vi "Properties to Property Info_2.vi"(6 "Class":string, 7 "Action":T1, 8 "Error In":errorcluster, 11 "All Properties for Refnum Terminal":T3(array[cluster])) -> (0 "Error Out":errorcluster, 2 "Properties for Tree Out":T2(array[cluster]), 3 "Property Info Array":T4(array[cluster]))   [LabVIEW 2023]
doc: "Take properties as returned by LabVIEW property node, and compile property info from property description file.\n\nThis version works for dialogs where you want to show the properties currently displayed in a node.e"
uses:
  controls/action enum.ctl
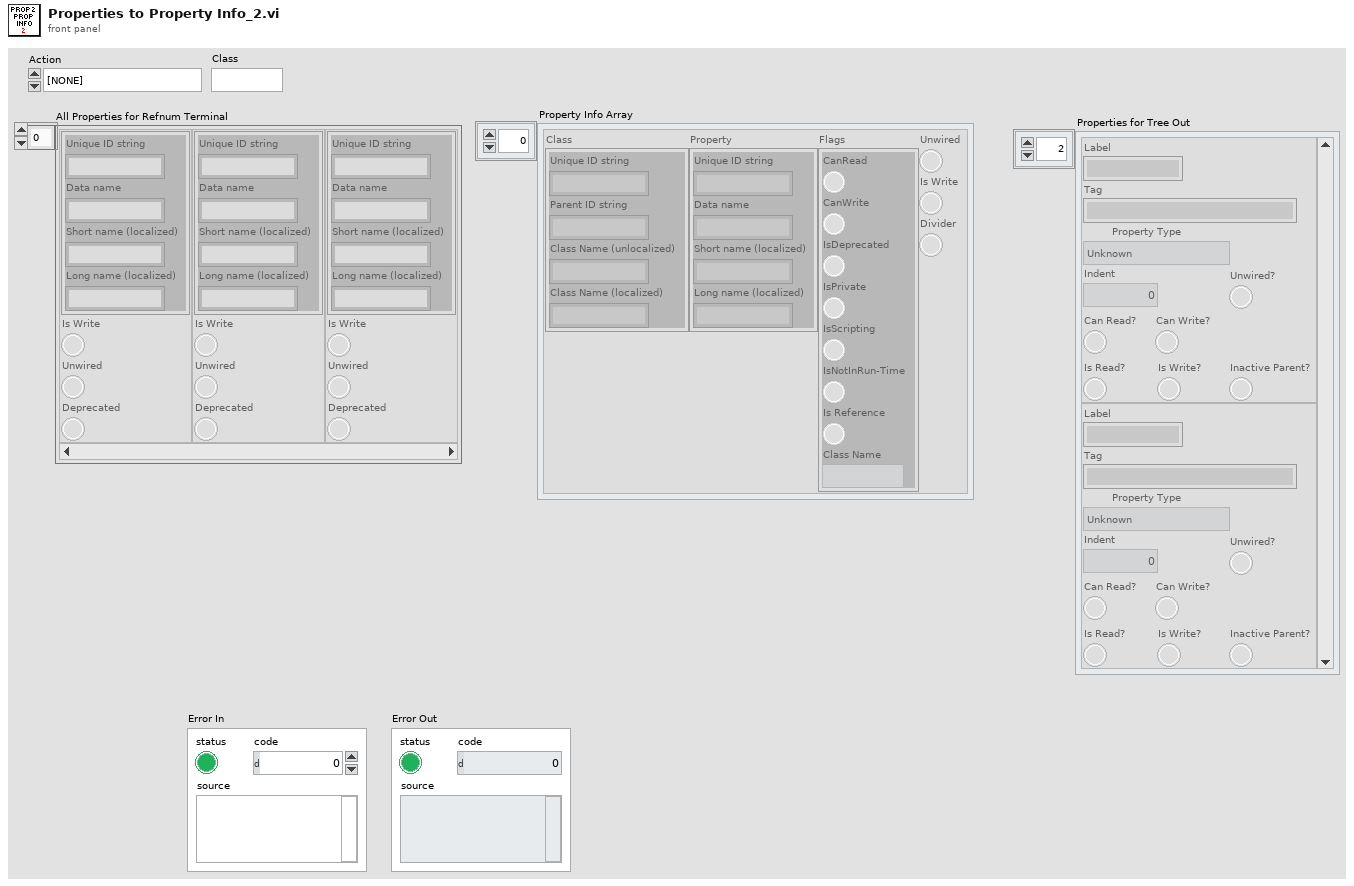
[diagram p1: front panel]
types:
  T1 = typedef "action enum.ctl" = enum16{"[NONE]", "Wire Bundle", "Wire Unbundle", "Terminal Unbundle", "Terminal Bundle", "Bundler Move Up", "Bundler Move Down", "Bundler Insert", "Bundler Remove", "Bundler Remove Unwired", "Bundler Rearrange", "In Place Insert", "In Place Remove", "In Place Remove Unwired", "In Place Rearrange", "Wire Properties", "Wire Method", "Terminal Properties", "Terminal Method", "Property Move Up", "Property Move Down", "Properties Insert", "Properties Remove", "Properties Remove Unwired", "Properties Rearrange", "Method Change", "Class for Constant", "Class For Control", "Class For Node", "Class Name to Clipboard"}
  T2 = cluster{"Label":string, "Tag":string, "Property Type":enum16{"Unknown", "Base", "Scripting", "Private", "Deprecated", "None", "Divider"}, "Indent":u16, "Can Read?":bool, "Can Write?":bool, "Is Read?":bool, "Is Write?":bool, "Inactive Parent?":bool, "Unwired?":bool}[]
  T3 = cluster{"Property/Method Info":cluster{"Unique ID string":string, "Data name":string, "Short name (localized)":string, "Long name (localized)":string}, "Is Write":bool, "Unwired":bool, "Deprecated":bool}[]
  T4 = cluster{"Class":cluster{"Unique ID string":string, "Parent ID string":string, "Class Name (unlocalized)":string, "Class Name (localized)":string}, "Property":cluster{"Unique ID string":string, "Data name":string, "Short name (localized)":string, "Long name (localized)":string}, "Flags":cluster{"CanRead":bool, "CanWrite":bool, "IsDeprecated":bool, "IsPrivate":bool, "IsScripting":bool, "IsNotInRun-Time":bool, "Is Reference":bool, "Class Name":string}, "Divider":bool, "Is Write":bool, "Unwired":bool}[]
  T5 = cluster{"Undotted Property":string, "Bare Property":string, "Is dotted?":bool, "Dot depth":i32, "Indent":i32, "Property Hierarchy":string[], "Parents":string[]}
  T6 = cluster{"Unique ID string":string, "Data name":string, "Short name (localized)":string, "Long name (localized)":string}
  T7 = cluster{"Class":cluster{"Unique ID string":string, "Parent ID string":string, "Class Name (unlocalized)":string, "Class Name (localized)":string}, "Property":cluster{"Unique ID string":string, "Data name":string, "Short name (localized)":string, "Long name (localized)":string}, "Flags":cluster{"CanRead":bool, "CanWrite":bool, "IsDeprecated":bool, "IsPrivate":bool, "IsScripting":bool, "IsNotInRun-Time":bool, "Is Reference":bool, "Class Name":string}, "Divider":bool, "Is Write":bool, "Unwired":bool}
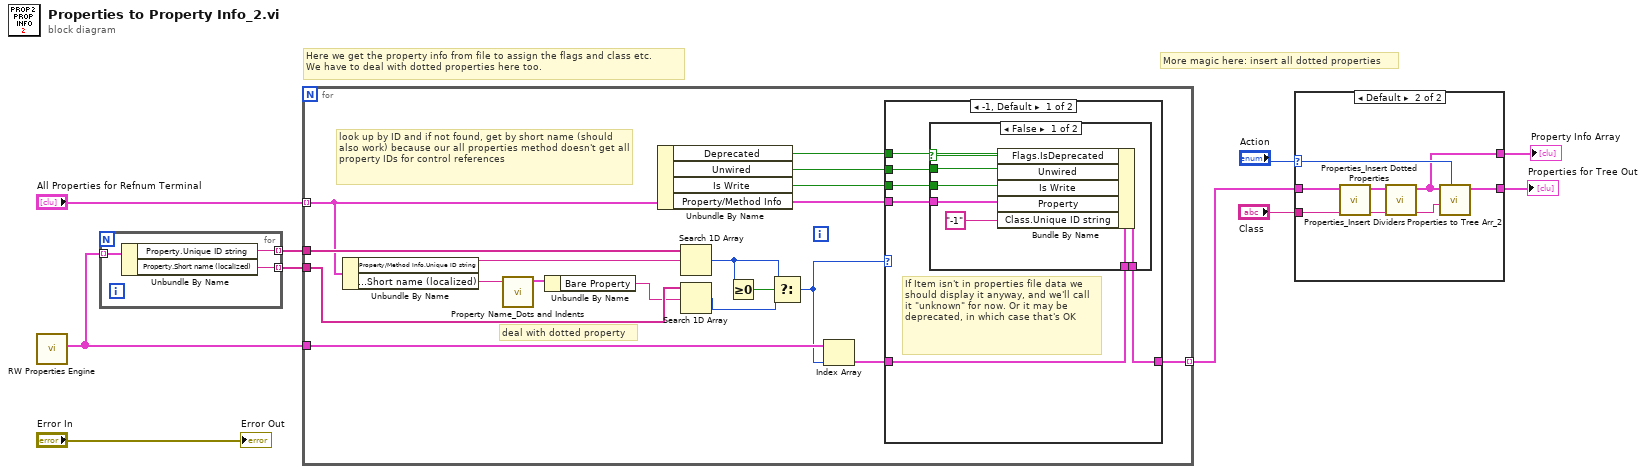
[diagram p0: block diagram]
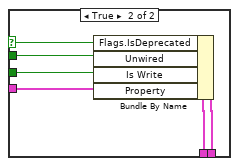
[diagram p2: hidden frame]
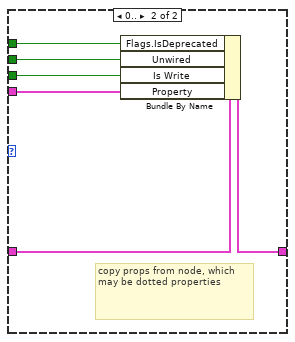
[diagram p3: hidden frame]
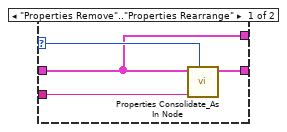
[diagram p4: hidden frame]
diagram:
  # "More magic here: insert all dotted properties"
  # "Here we get the property info from file to assign the flags and class etc. \nWe have to deal with dotted properties here too."
  n1 = call "RW Properties Engine.vi"() -> ("Properties Out"=w10:T4)  [unwired: 7 in, 4 out]
  n2 = for {
    tunnel: w10 -> [w13] mode=indexing
    tunnel: [w12] -> w8 mode=indexing
    tunnel: [w11] -> w7 mode=indexing
    n3 = Unbundle By Name(w13) -> ("Property.Unique ID string"=w12:string, "Property.Short name (localized)"=w11:string)
  }
  n4 = for {
    tunnel: w8 -> [w31]
    tunnel: "All Properties for Refnum Terminal" -> [w14] mode=indexing
    tunnel: w10 -> [w29]
    tunnel: [w27] -> w2 mode=indexing
    tunnel: w7 -> [w26]
    # "deal with dotted property"
    # "look up by ID and if not found, get by short name (should also work) because our all properties method doesn't get all property IDs for control references"
    n5 = Unbundle By Name(w14) -> ("Property/Method Info.Unique ID string"=w30:string, "Property/Method Info.Short name (localized)"=w21:string)
    n6 = call "Property Name_Dots and Indents.vi"("Property"=w21) -> ("Cluster"=w20:T5)  [unwired: 10 in]
    n7 = Unbundle By Name(w20) -> ("Bare Property"=w19:string)
    n8 = Unbundle By Name(w14) -> ("Deprecated"=w15:bool, "Unwired"=w17:bool, "Is Write"=w16:bool, "Property/Method Info"=w18:T6)
    n9 = Search 1D Array(1D array=w31, element=w30) -> (index of element=w23:i32)  [unwired: 1 in]
    n10 = Search 1D Array(1D array=w26, element=w19) -> (index of element=w24:i32)  [unwired: 1 in]
    n11 = Greater Or Equal To 0?(x=w23) -> (x >= 0?=w25:bool)
    n12 = Select(t=w23, s=w25, f=w24) -> (s? t:f=w22:i32)
    n13 = Index Array(array=w29, index=w22) -> (element=w28:T7)
    n14 = case shown="-1, Default" w22 {
      tunnel: [w37 w56] -> w27
      tunnel: w28 -> [w34 w55]
      tunnel: w18 -> [w33 w54]
      tunnel: w17 -> [w36 w53]
      tunnel: w16 -> [w35 w52]
      tunnel: w15 -> [w32 w51]
      frame -1, Default {
        # "If Item isn't in properties file data we should display it anyway, and we'll call it \"unknown\" for now. Or it may be deprecated, in which case that's OK"
        n15 = case shown="False" w32 {
          selector: w32 -> [w38 w45]
          tunnel: [w44 w50] -> w37
          tunnel: w36 -> [w43 w49]
          tunnel: w35 -> [w42 w48]
          tunnel: w34 -> [w41 w47]
          tunnel: w33 -> [w40 w46]
          frame False {
            n16 = Bundle By Name(cluster=w41, "Flags.IsDeprecated"=w38, "Unwired"=w43, "Is Write"=w42, "Property"=w40, "Class.Unique ID string"="-1" ("Class Info.Unique ID string")) -> (w44:T7)
          }
          frame True {
            n17 = Bundle By Name(cluster=w47, "Flags.IsDeprecated"=w45, "Unwired"=w49, "Is Write"=w48, "Property"=w46) -> (w50:T7)
          }
        }
      }
      frame 0.. {
        # "copy props from node, which may be dotted properties"
        n18 = Bundle By Name(cluster=w55, "Flags.IsDeprecated"=w51, "Unwired"=w53, "Is Write"=w52, "Property"=w54) -> (w56:T7)
      }
    }
  }
  n19 = case shown="Default" "Action" {
    selector: "Action" -> [w59 w65]
    tunnel: [w60 w66] -> w6
    tunnel: w2 -> [w57 w62]
    tunnel: "Class" -> [w58 w64]
    tunnel: [w57 w63] -> w1
    frame "Properties Remove".."Properties Rearrange" {
      n20 = call "Properties Consolidate_As In Node.vi"("Action"=w59, "Class"=w58, "Property Info Array"=w57) -> ("Property Info Out"=w60:T2)  [unwired: 8 in]
    }
    frame Default {
      n21 = call "Properties_Insert Dividers.vi"("Property Info Array In"=w62) -> ("Property Info Array Out"=w61:T4)  [unwired: 9 in, 1 out]
      n22 = call "Properties_Insert Dotted Properties.vi"("Property Info Array In"=w61) -> ("Property Info Array Out"=w63:T4)  [unwired: 8 in, 2 out]
      n23 = call "Properties to Tree Arr_2.vi"("Action"=w65, "Class"=w64, "Properties In"=w63) -> ("Properties for Tree Out"=w66:T2)  [unwired: 8 in]
    }
  }
  "Property Info Array" <- w1
  "Properties for Tree Out" <- w6
  "Error Out" <- "Error In"
